vi "LCC Get No Of Control Channels.vi"(8 "error in (no error)":errorcluster caption="Fehler (Eingang, kein Fehler)") -> (0 "error out":errorcluster caption="Fehler (Ausgang)", 3 "Control Channel Count":i32)   [LabVIEW 2021, in "labbCAN_Controller_API.lvlib"]
doc: "LCC_Func long LCC_CALL LCC_GetNoOfControlChannels();"
uses:
  labbCAN_Controller_API.lvlib
  labbCAN_Controller_API.dll
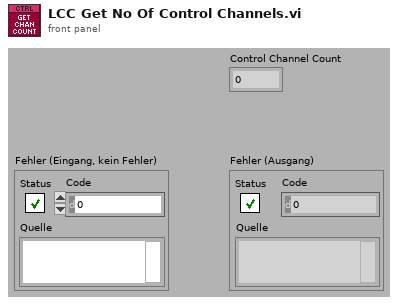
[diagram p1: front panel]
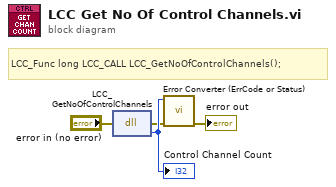
[diagram p0: block diagram]
diagram:
  # "LCC_Func long LCC_CALL LCC_GetNoOfControlChannels();"
  n1 = dll-call lib="C:/Users/olaja/AppData/Local/CETONI_SDK/labbCAN_Controller_API.*" fn="LCC_GetNoOfControlChannels"(error in="error in (no error)") -> (error out=w2:errorcluster, "Rückgabetyp"=w4:i32)  [unwired: 2 in, 1 out]
  "Control Channel Count" <- w4
  n2 = call "Error Converter (ErrCode or Status).vi"("error in (no error)"=w2, "error code"=w4) -> ("error out"=→"error out":errorcluster)  [unwired: 9 in]
